vi "Load_Info.vi"(8 "error in (no error)":errorcluster, 11 "AB_Targetfile in":refnum<class "AB_Targetfile.lvclass">) -> (0 "error out":errorcluster, 3 "AB_Targetfile out":refnum<class "AB_Targetfile.lvclass">)   [LabVIEW 2020, in "AB_Targetfile.lvclass"]
uses:
  <vilib>/AppBuilder/AB_Classes/TargetFile/AB_Targetfile.lvclass
  e:/builds/penguin/labview/branches/2020/dev/dist/vi.lib/AppBuilder/AB_Classes/Build/AB_Build.lvclass
  <vilib>/AppBuilder/RW_Project/AB_RW_Project_PropBag_Action.ctl
  <vilib>/AppBuilder/AB_Classes/TargetFile/AB_Targetfile.lvclass/AB_Targetfile.ctl
  <vilib>/AppBuilder/AB_Classes/Build/AB_Build.lvclass
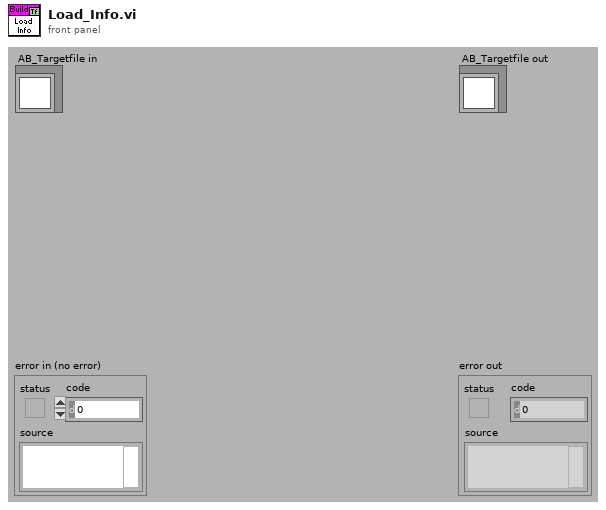
[diagram p1: front panel]
types:
  T1 = typedef "AB_RW_Project_PropBag_Action.ctl" = enum16{"read", "write", "clear", "readPrevious", "writePrevious", "clearPrevious"}
  T2 = typedef "AB_Build.ctl" = cluster{"buildSpecName":string, "buildSpecDescription":string, "destinations":refnum<class "AB_Destination.lvclass">[], "exclusionOption":T3, "defaultLanguage":string, "supportedLanguages":string[], "excludedDirectories":path[], "buildContext":refnum<vi>, "buildObject":T4, "preview":bool, "programatic":bool, "progressBarEvents":T5, "userLog_Path":path, "preActionID":string, "preAction_Path":path, "postActionID":string, "postAction_Path":path, "eng_checkForBrokenVIs?":bool, "eng_verboseLinkerErrors?":bool, "localDest_Path":path, "targetDest_Path":path, "removeVIObject":u16, "cache":refnum<class "PreviewCache.lvclass">, "use cache":bool, "previewCache_ID":string, "buildCache_ID":string, "eng_TempLocalDest_Path":path, "eng_collectDependencies?":bool, "versionInfo":cluster{"buildVersion":cluster{"major":u16, "minor":u16, "patch":u16, "build":u16}, "autoIncrement":bool}, "eng_enableVIChecksums":bool}
  T3 = typedef "AB_Exclusion_Option.ctl" = cluster{"typedefs":bool, "polymorphicVIs":bool, "unusedLibraryItems":bool, "modifyLibraryFile":bool, "edit-timeDependencies":bool, "inlineVIs":bool, "dependent PPLs":bool, "dependent DLLs":bool}
  T4 = typedef "ItemRef.ctl" = u64
  T5 = typedef "provcom_ProgressBar_Events.ctl" = cluster{"newJob":refnum<user-event>, "newItem":refnum<user-event>, "errorMsg":T6, "cancel":refnum<user-event>}
  T6 = typedef "mxLvBuildError.ctl" = refnum<user-event>
  T7 = typedef "AB_RW_Project_TargetFile_Data.ctl" = cluster{"targetfileName":string, "targetfileGUID":string, "enableDebugging":bool, "productName":string, "legalCopyright":string, "companyName":string, "internalName":string, "fileDescription":string, "eng_topLevelVI_DestinationPaths":path[], "fastFileFormat":bool, "versionIndependent":bool}
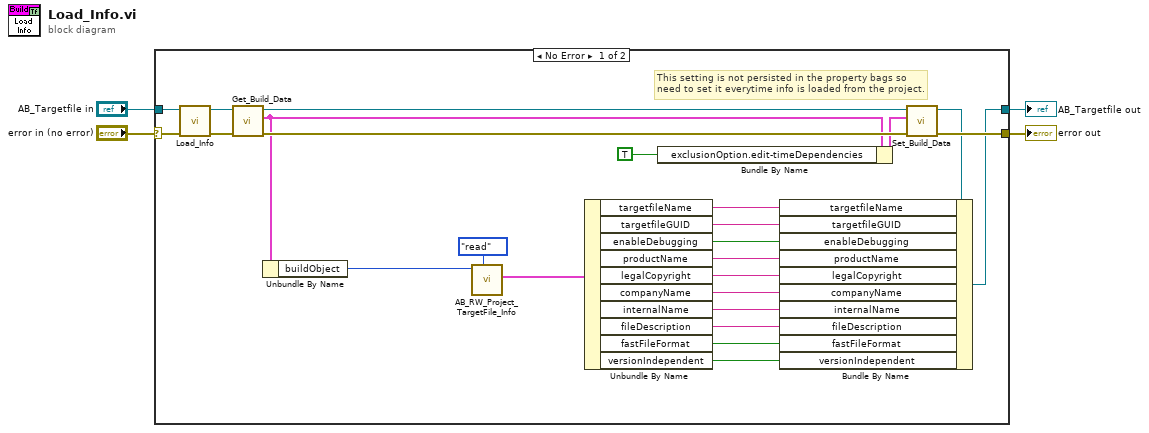
[diagram p0: block diagram]
diagram:
  n1 = case shown="No Error" "error in (no error)" {
    selector: "error in (no error)" -> [w28 w30]
    tunnel: [w22 w30] -> w4
    tunnel: [w16 w31] -> w3
    tunnel: "AB_Targetfile in" -> [w29 w31]
    frame No Error {
      # "This setting is not persisted in the property bags so need to set it everytime info is loaded from the project."
      n2 = call-parent "Load_Info.vi"("error in (no error)"=w28, "AB_Build in"=w29) -> ("error out"=w23:errorcluster, "AB_Build out"=w27:refnum<class "AB_Targetfile.lvclass">)  [unwired: 8 in]
      n3 = call <vilib>:"Get_Build_Data.vi"("error in (no error)"=w23, "Class in"=w27) -> ("error out"=w24:errorcluster, "data"=w21:T2, "Class out"=w25:refnum<class "AB_Targetfile.lvclass">)  [unwired: 7 out]
      n4 = Unbundle By Name(w21) -> ("buildObject"=w19:T4)
      n5 = call <vilib>:"AB_RW_Project_TargetFile_Info.vi"("action"=AB_RW_Project_PropBag_Action."read", "Object In"=w19) -> ("targetfile info"=w17:T7)  [unwired: 7 in, 2 out]
      n6 = Unbundle By Name(w17) -> ("targetfileName"=w14:string, "targetfileGUID"=w13:string, "enableDebugging"=w12:bool, "productName"=w11:string, "legalCopyright"=w10:string, "companyName"=w9:string, "internalName"=w8:string, "fileDescription"=w7:string, "fastFileFormat"=w6:bool, "versionIndependent"=w5:bool)
      n7 = Bundle By Name(cluster=w21, "exclusionOption.edit-timeDependencies"=TRUE) -> (w20:T2)
      n8 = call <vilib>:"Set_Build_Data.vi"("error in (no error)"=w24, "data"=w20, "Class in"=w25) -> ("error out"=w22:errorcluster, "Class out"=w15:refnum<class "AB_Targetfile.lvclass">)  [unwired: 7 out]
      n9 = Bundle By Name(cluster=w15, "targetfileName"=w14, "targetfileGUID"=w13, "enableDebugging"=w12, "productName"=w11, "legalCopyright"=w10, "companyName"=w9, "internalName"=w8, "fileDescription"=w7, "fastFileFormat"=w6, "versionIndependent"=w5) -> (w16:refnum<class "AB_Targetfile.lvclass">)
    }
    frame Error {
    }
  }
  "error out" <- w4
  "AB_Targetfile out" <- w3
